vi "Periodic Tasks.vi"() -> ()   [LabVIEW 2011]
doc: "This VI runs in parallel to other tasks. It can contain as many user-defined periodic loops as you need. These can carry out PID or other sorts of timed response."
uses:
  <vilib>/Rock Robotics/SystemInterfaces/Utilities/FPGA_UtilitiesLED State.ctl
  <vilib>/Rock Robotics/SystemInterfaces/Utilities/FPGA_UtilitiesLED Source.ctl
  Robot Global Data.vi
  <vilib>/Rock Robotics/WPI/Relay/WPI_RelayValue.ctl
panel:
  out "Both Hit?":bool
  out "Desired Ramp POT Voltage":dbl
  out "Ramp POT Angle":dbl
  out "Ramp Pot Voltage":dbl
  out "ON/OFF":bool
  out "Rate 3":dbl
  out "error out 4":errorcluster
  out "Direction 3":bool
  out "Distance 3":dbl
  out "Distance 2":dbl
  out "Direction 2":bool
  out "error out 3":errorcluster
  out "Rate 2":dbl
  out "Rate":dbl
  out "error out 2":errorcluster
  out "I2C":bool
  out "Angular Rate":dbl
  out "Angle":dbl
  out "Direction":bool
  out "Distance":dbl
  # "Speed to move to home"
  # "Target Tracking"
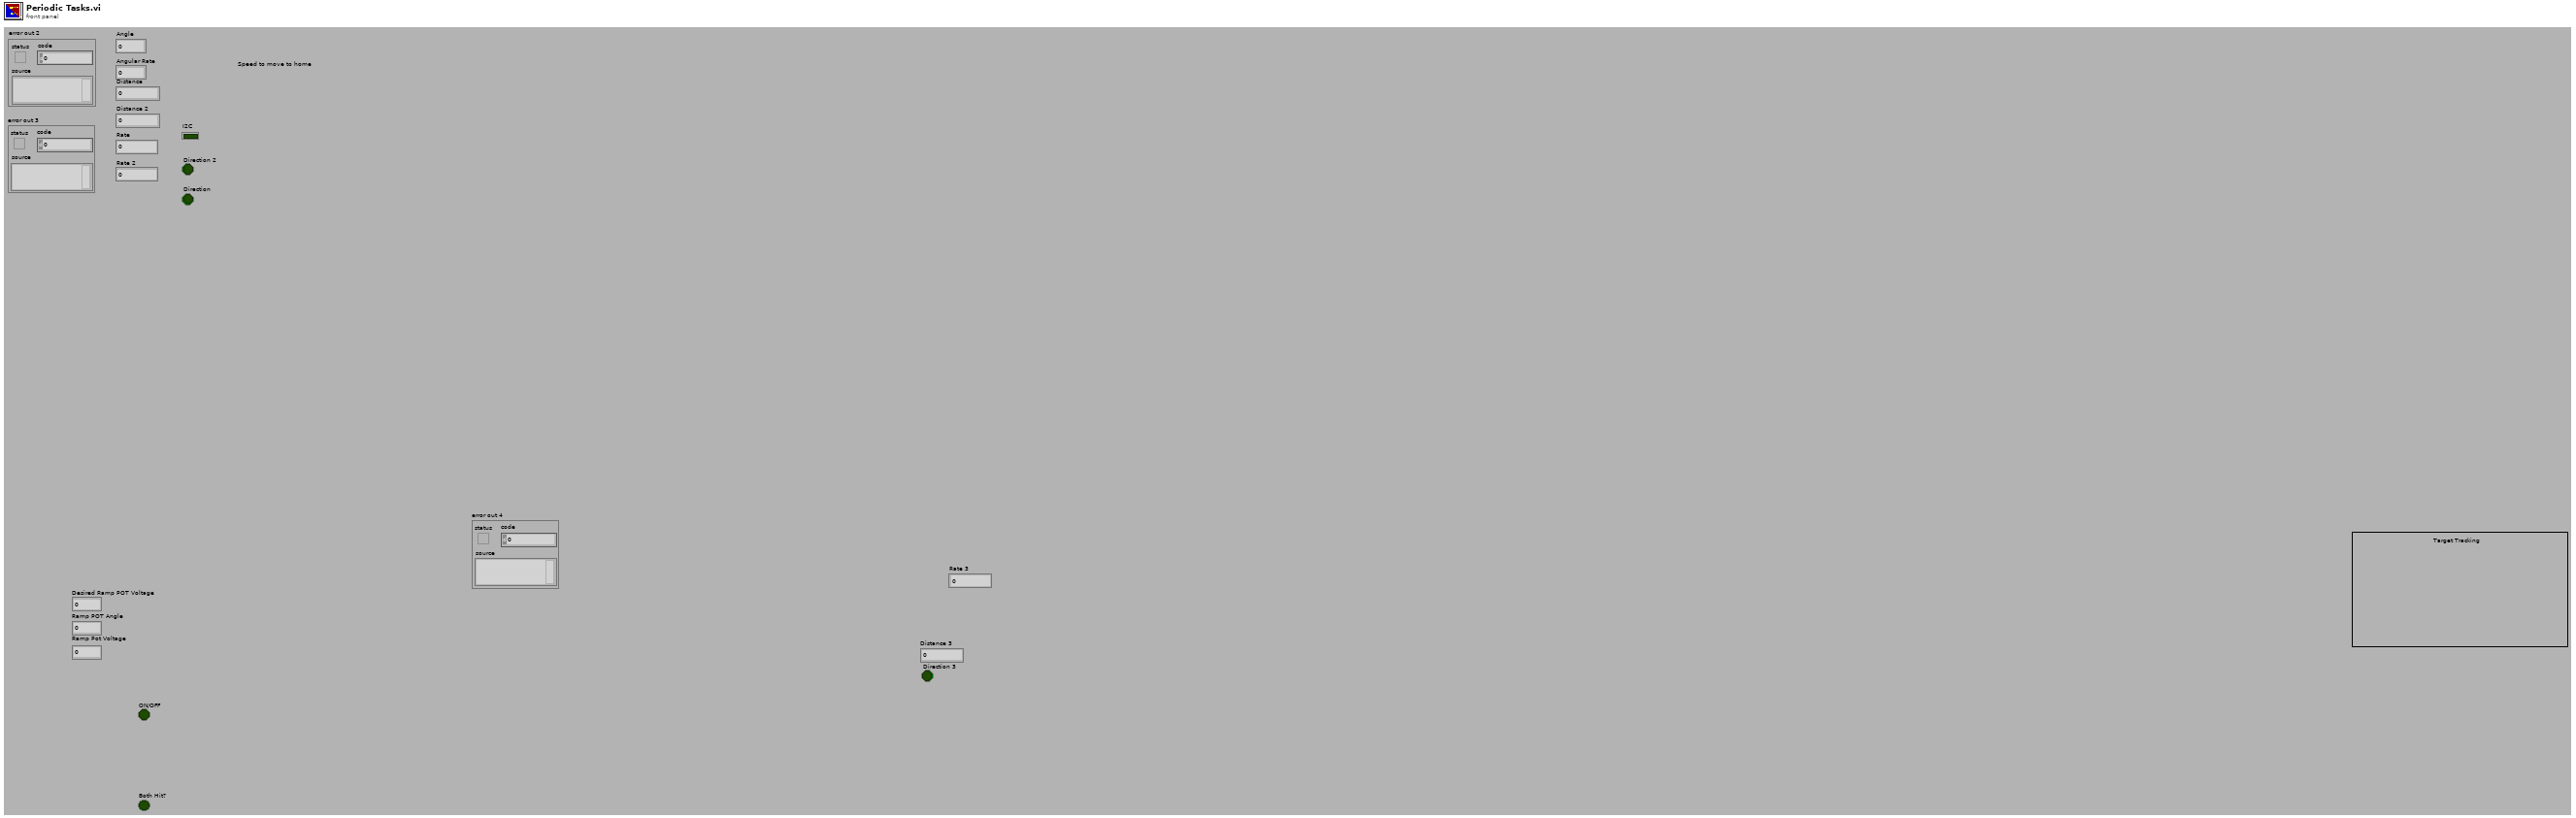
[diagram p1: front panel]
types:
  T1 = typedef "WPI_EncoderDevRef.ctl" = cluster{"DevStatus":errorcluster, "EncoderIndex":T2, "CounterIndex":T3, "DistancePerCount":dbl, "Decoding Type":T4}
  T2 = typedef "FPGA_EncoderIdx.ctl" = enum8{"Enc 0", "Enc 1", "Enc 2", "Enc 3", "Invalid"}
  T3 = typedef "FPGA_CounterCtrSystemIndex.ctl" = enum8{"Ctr 0", "Ctr 1", "Ctr 2", "Ctr 3", "Ctr 4", "Ctr 5", "Ctr 6", "Ctr 7", "Invalid"}
  T4 = typedef "WPI_EncoderType.ctl" = enum16{"1x", "2x", "4x"}
  T5 = typedef "WPI_RelayValue.ctl" = enum16{"Off", "On", "Forward", "Reverse"}
  T6 = typedef "WPI_AnalogChannelDevRef.ctl" = cluster{"DevStatus":errorcluster, "Analog Module":T7, "Analog Channel":T8}
  T7 = typedef "FPGA_TypedefAnalogModule.ctl" = enum16{"Analog Module 1", "Analog Module 2"}
  T8 = typedef "FPGA_AIChannel.ctl" = enum8{"AI 1", "AI 2", "AI 3", "AI 4", "AI 5", "AI 6", "AI 7", "AI 8", "Invalid"}
  T9 = typedef "WPI_RelayDevRef.ctl" = cluster{"DevStatus":errorcluster, "Relay Channel":T10, "Digital Module":T11, "Relay Direction":T12}
  T10 = typedef "FPGA_DIORelayChannel.ctl" = enum8{"Relay 1", "Relay 2", "Relay 3", "Relay 4", "Relay 5", "Relay 6", "Relay 7", "Relay 8", "Invalid"}
  T11 = typedef "FPGA_TypedefDigitalModule.ctl" = enum16{"Digital Module 1", "Digital Module 2"}
  T12 = typedef "WPI_RelayDirection.ctl" = enum16{"Both directions", "Forward only", "Reverse only"}
  T13 = typedef "WPI_GyroDevRef.ctl" = cluster{"DevStatus":errorcluster, "Analog Module":T7, "Analog Channel":T8, "Offset":dbl, "Gain (VoltsPerDegree/Second)":dbl}
  T14 = typedef "WPI_JoystickDevRef.ctl" = cluster{"Device":T15}
  T15 = typedef "WPI_JoystickDeviceEnum.ctl" = enum16{"USB 1", "USB 2", "USB 3", "USB 4", "Kinect 1", "Kinect 2"}
  T16 = cluster{"axis 1 (x)":dbl, "axis 2 (y)":dbl, "axis 3 (throttle)":dbl, "axis 4":dbl, "axis 5":dbl, "axis 6":dbl}
  T17 = typedef "WPI_JoystickButtonState.ctl" = cluster{"Button 1":bool, "Button 2":bool, "Button 3":bool, "Button 4":bool, "Button 5":bool, "Button 6":bool, "Button 7":bool, "Button 8":bool, "Button 9":bool, "Button 10":bool, "Button 11":bool, "Button 12":bool}
  T18 = typedef "WPI_MotorControlDeviceRef.ctl" = cluster{"DeviceStatus":errorcluster, "Type":enum16{"PWM", "CAN"}, "PWM":cluster{"Digital Module":T11, "PWM Channel":T19, "DeadBand":T20}, "CAN":cluster{"Device Number":u8, "Control Mode":T21, "Semaphore":T22, "Max Vout":dbl}, "Invert":bool, "TransformRef":T23, "InvTransformRef":T23}
  T19 = typedef "FPGA_DIOPWMChannel.ctl" = enum8{"PWM 1", "PWM 2", "PWM 3", "PWM 4", "PWM 5", "PWM 6", "PWM 7", "PWM 8", "PWM 9", "PWM 10", "Invalid"}
  T20 = typedef "WPI_PWMDeadband.ctl" = cluster{"Name":string, "maxPositivePwm":i32, "minPositivePwm":i32, "centerPwm":i32, "maxNegativePwm":i32, "minNegativePwm":i32, "angularRange":u16}
  T21 = typedef "WPI_CANJaguar_ControlMode.ctl" = enum8{"Percent VBus", "Current", "Speed", "Position", "Voltage"}
  T22 = typedef "Semaphore RefNum" = refnum<k1>
  T23 = typedef "WPI_PWMTransform_ConPane.ctl" = refnum<vi>
  T24 = cluster{"Driver Station Digital Output (1-8)[0]":bool, "Driver Station Digital Output (1-8)[1]":bool, "Driver Station Digital Output (1-8)[2]":bool, "Driver Station Digital Output (1-8)[3]":bool, "Driver Station Digital Output (1-8)[4]":bool, "Driver Station Digital Output (1-8)[5]":bool, "Driver Station Digital Output (1-8)[6]":bool, "Driver Station Digital Output (1-8)[7]":bool, "Driver Station Digital Output (1-8)[8]":bool}
  T25 = typedef "FPGA_UtilitiesLED State.ctl" = enum16{"Off", "On", "Toggle"}
  T26 = typedef "FPGA_UtilitiesLED Source.ctl" = enum16{"User LED", "FPGA LED"}
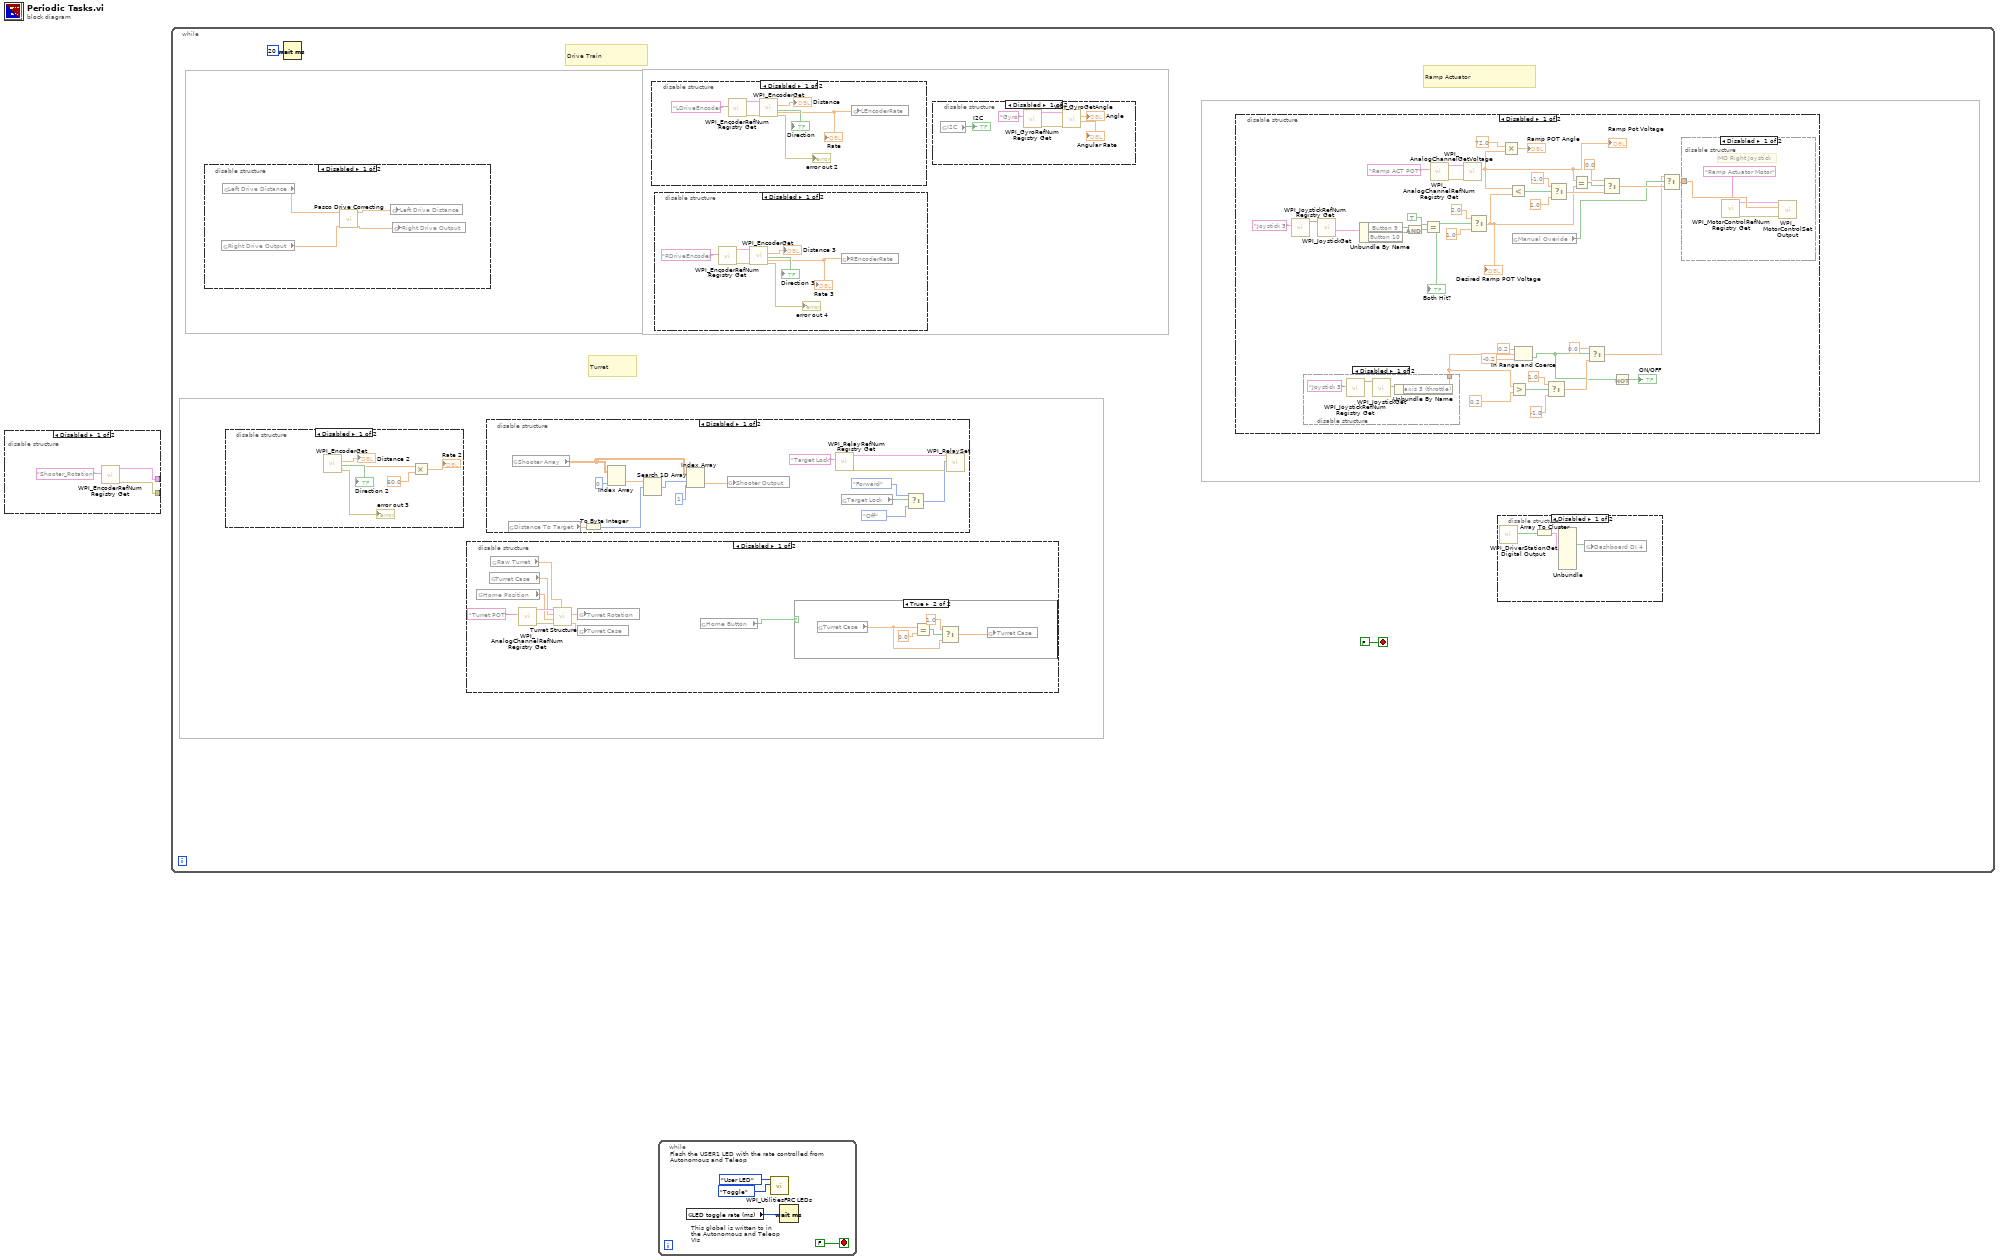
[diagram p0: block diagram]
diagram:
  n1 = disable-structure shown="Disabled" {
    disable-tunnel: [w2 _] -> _
    disable-tunnel: [w1 _] -> _
    frame Disabled {
      n2 = call <vilib>:"WPI_EncoderRefNum Registry Get.vi"("refnum name"="Shooter_Rotation") -> ("error out"=w2:errorcluster, "EncoderDevRef"=w1:T1)  [unwired: 9 in]
    }
    frame Enabled {
    }
  }
  n3 = while {
    stop <- FALSE stop-if-true
    # "Turret"
    # "Drive Train"
    # "Ramp Actuator"
    n4 = disable-structure shown="Disabled" {
      frame Disabled {
        n5 = global read "Robot Global Data.vi" "Right Drive Output"() -> (w8:dbl)
        n6 = global read "Robot Global Data.vi" "Left Drive Distance"() -> (w9:dbl)
        n7 = call "Pasco Drive Correcting.vi"("RightDriveOutput"=w8, "LeftDriveOutput"=w9) -> ("RightDriveOutput"=w6:dbl, "LeftDriveOutput"=w7:dbl)  [unwired: 8 in]
        n8 = global write "Robot Global Data.vi" "Left Drive Distance"(w7) -> ()
        n9 = global write "Robot Global Data.vi" "Right Drive Output"(w6) -> ()
      }
      frame Enabled {
      }
    }
    n10 = disable-structure shown="Disabled" {
      frame Disabled {
        n11 = call <vilib>:"WPI_EncoderGet.vi"() -> ("error out"=→"error out 3":errorcluster, "Direction"=→"Direction 2":bool, "Distance"=→"Distance 2":dbl, "Rate"=w94:dbl)  [unwired: 6 in, 2 out]
        n12 = Multiply(x=w94, y=60.0) -> (x*y=→"Rate 2":dbl)
      }
      frame Enabled {
      }
    }
    n13 = Wait (ms)(milliseconds to wait=u32 20) -> ()  [unwired: 1 out]
    n14 = disable-structure shown="Disabled" {
      frame Disabled {
        n15 = global read "Robot Global Data.vi" "Home Position"() -> (w17:dbl)
        n16 = global read "Robot Global Data.vi" "Turret Case"() -> (w18:dbl)
        n17 = global read "Robot Global Data.vi" "Raw Turret"() -> (w16:dbl)
        n18 = call <vilib>:"WPI_AnalogChannelRefNum Registry Get.vi"("refnum name"="Turret POT") -> ("error out"=w19:errorcluster, "AIDeviceRef"=w20:T6)  [unwired: 9 in]
        n19 = call "Turret Structure.vi"("Raw Turret"=w16, "error in (no error)"=w19, "Home postion"=w17, "Turret Case"=w18, "AIDeviceRef"=w20) -> ("Turret Case Output"=w14:dbl, "Turret Output"=w15:dbl)  [unwired: 5 in]
        n20 = global write "Robot Global Data.vi" "Turret Rotation"(w15) -> ()
        n21 = global write "Robot Global Data.vi" "Turret Case"(w14) -> ()
        n22 = global read "Robot Global Data.vi" "Home Button"() -> (w13:bool)
        n23 = case shown="True" w13 {
          frame False {
          }
          frame True {
            n24 = global read "Robot Global Data.vi" "Turret Case"() -> (w23:dbl)
            n25 = Equal?(x=w23, y=0.0) -> (x = y?=w25:bool)
            n26 = Select(t=1.0, s=w25, f=w23) -> (s? t:f=w22:dbl)
            n27 = global write "Robot Global Data.vi" "Turret Case"(w22) -> ()
          }
        }
      }
      frame Enabled {
      }
    }
    n28 = disable-structure shown="Disabled" {
      frame Disabled {
        n29 = global read "Robot Global Data.vi" "Distance To Target"() -> (w104:dbl)
        n30 = global read "Robot Global Data.vi" "Shooter Array"() -> (w102:dbl[][])
        n31 = To Byte Integer(number=w104) -> (8bit integer=w103:i8)
        n32 = Index Array(array=w102, index (col)=0 ("disabled index (col)")) -> (element=w105:dbl[])  [unwired: 1 in]
        n33 = Search 1D Array(1D array=w105, element=w103) -> (index of element=w101:i32)  [unwired: 1 in]
        n34 = Index Array(array=w102, index (row)=w101, index (col)=1 ("disabled index (col)")) -> (element=w99:dbl)
        n35 = global write "Robot Global Data.vi" "Shooter Output"(w99) -> ()
        n36 = call <vilib>:"WPI_RelayRefNum Registry Get.vi"("refnum name"="Target Lock") -> ("error out"=w107:errorcluster, "RelayDevRef"=w108:T9)  [unwired: 9 in]
        n37 = global read "Robot Global Data.vi" "Target Lock"() -> (w113:bool)
        n38 = Select(t=WPI_RelayValue."Forward" ("RelayValue"), s=w113, f=WPI_RelayValue."Off" ("RelayValue")) -> (s? t:f=w110:T5)
        n39 = call <vilib>:"WPI_RelaySet.vi"("error in (no error)"=w107, "RelayValue"=w110, "RelayDevRef"=w108) -> ()  [unwired: 7 in, 2 out]
      }
      frame Enabled {
      }
    }
    n40 = disable-structure shown="Disabled" {
      frame Disabled {
        n41 = call <vilib>:"WPI_EncoderRefNum Registry Get.vi"("refnum name"="LDriveEncoder") -> ("error out"=w84:errorcluster, "EncoderDevRef"=w83:T1)  [unwired: 9 in]
        n42 = call <vilib>:"WPI_EncoderGet.vi"("error in (no error)"=w84, "EncoderDevRef"=w83) -> ("error out"=→"error out 2":errorcluster, "Direction"=→"Direction":bool, "Distance"=→"Distance":dbl, "Rate"=w80:dbl)  [unwired: 4 in, 2 out]
        "Rate" <- w80
        n43 = global write "Robot Global Data.vi" "LEncoderRate"(w80) -> ()
      }
      frame Enabled {
      }
    }
    n44 = disable-structure shown="Disabled" {
      frame Disabled {
        n45 = call <vilib>:"WPI_EncoderRefNum Registry Get.vi"("refnum name"="RDriveEncoder") -> ("error out"=w77:errorcluster, "EncoderDevRef"=w76:T1)  [unwired: 9 in]
        n46 = call <vilib>:"WPI_EncoderGet.vi"("error in (no error)"=w77, "EncoderDevRef"=w76) -> ("error out"=→"error out 4":errorcluster, "Direction"=→"Direction 3":bool, "Distance"=→"Distance 3":dbl, "Rate"=w73:dbl)  [unwired: 4 in, 2 out]
        "Rate 3" <- w73
        n47 = global write "Robot Global Data.vi" "REncoderRate"(w73) -> ()
      }
      frame Enabled {
      }
    }
    n48 = disable-structure shown="Disabled" {
      frame Disabled {
        n49 = global read "Robot Global Data.vi" "I2C"() -> (→"I2C":bool)
        n50 = call <vilib>:"WPI_GyroRefNum Registry Get.vi"("refnum name"="Gyro") -> ("error out"=w91:errorcluster, "GyroDevRef"=w92:T13)  [unwired: 9 in]
        n51 = call <vilib>:"WPI_GyroGetAngle.vi"("error in (no error)"=w91, "GyroDevRef"=w92) -> ("Angular Rate"=→"Angular Rate":dbl, "Angle"=→"Angle":dbl)  [unwired: 6 in, 2 out]
      }
      frame Enabled {
      }
    }
    n52 = disable-structure shown="Disabled" {
      frame Disabled {
        n53 = call <vilib>:"WPI_JoystickRefNum Registry Get.vi"("refnum name"="Joystick 3") -> ("JoystickDevRef"=w62:T14)  [unwired: 9 in, 1 out]
        n54 = disable-structure shown="Disabled" {
          disable-tunnel: [w69 _] -> w33
          frame Disabled {
            n55 = call <vilib>:"WPI_JoystickRefNum Registry Get.vi"("refnum name"="Joystick 3") -> ("JoystickDevRef"=w72:T14)  [unwired: 9 in, 1 out]
            n56 = call <vilib>:"WPI_JoystickGet.vi"("JoystickDevRef"=w72) -> ("Axes"=w70:T16)  [unwired: 4 in, 2 out]
            n57 = Unbundle By Name(w70) -> ("axis 3 (throttle)"=w69:dbl)
          }
          frame Enabled {
          }
        }
        n58 = call <vilib>:"WPI_JoystickGet.vi"("JoystickDevRef"=w62) -> ("Buttons"=w64:T17)  [unwired: 4 in, 2 out]
        n59 = Unbundle By Name(w64) -> ("Button 9"=w61:bool, "Button 10"=w60:bool)
        n60 = And(x=w61, y=w60) -> (x .and. y?=w59:bool)
        n61 = Equal?(x=TRUE, y=w59) -> (x = y?=w54:bool)
        "Both Hit?" <- w54
        n62 = call <vilib>:"WPI_AnalogChannelRefNum Registry Get.vi"("refnum name"="Ramp ACT POT") -> ("error out"=w57:errorcluster, "AIDeviceRef"=w56:T6)  [unwired: 9 in]
        n63 = call <vilib>:"WPI_AnalogChannelGetVoltage.vi"("error in (no error)"=w57, "AIDeviceRef"=w56) -> ("Voltage"=w44:dbl)  [unwired: 7 in, 2 out]
        "Ramp Pot Voltage" <- w44
        n64 = Select(t=2.0, s=w54, f=1.0 ("t")) -> (s? t:f=w47:dbl)
        "Desired Ramp POT Voltage" <- w47
        n65 = Multiply(x=72.0, y=w44) -> (x*y=→"Ramp POT Angle":dbl)
        n66 = Less?(x=w44, y=w47) -> (x < y?=w51:bool)
        n67 = Greater?(x=w33, y=0.2) -> (0:w34:bool)
        n68 = global read "Robot Global Data.vi" "Manual Overide"() -> (w40:bool)
        n69 = In Range and Coerce(upper limit=0.2, x=w33, lower limit=-0.2) -> (In Range?=w28:bool)  [unwired: 1 out]
        n70 = Select(t=1.0, s=w34, f=-1.0) -> (s? t:f=w35:dbl)
        n71 = Select(t=-1.0, s=w51, f=1.0) -> (s? t:f=w50:dbl)
        n72 = Equal?(x=w44, y=w47) -> (x = y?=w53:bool)
        n73 = Select(t=0.0, s=w28, f=w35) -> (s? t:f=w29:dbl)
        n74 = Select(t=0.0, s=w53, f=w50) -> (s? t:f=w41:dbl)
        n75 = Not(x=w28) -> (.not. x?=→"ON/OFF":bool)
        n76 = Select(t=w29, s=w40, f=w41) -> (s? t:f=w39:dbl)
        n77 = disable-structure shown="Disabled" {
          disable-tunnel: w39 -> [w67 _]
          frame Disabled {
            # "MO Right Joystick"
            n78 = call <vilib>:"WPI_MotorControlRefNum Registry Get.vi"("refnum name"="Ramp Actuator Motor") -> ("error out"=w68:errorcluster, "MotorControlDevRef"=w66:T18)  [unwired: 9 in]
            n79 = call <vilib>:"WPI_MotorControlSetOutput.vi"("error in (no error)"=w68, "Output"=w67, "MotorControlDevRef"=w66) -> ()  [unwired: 7 in, 2 out]
          }
          frame Enabled {
          }
        }
      }
      frame Enabled {
      }
    }
    n80 = disable-structure shown="Disabled" {
      frame Disabled {
        n81 = call <vilib>:"WPI_DriverStationGet Digital Output.vi"() -> ("Driver Station Digital Output (1-8)"=w12:bool[])  [unwired: 10 in, 1 out]
        n82 = Array To Cluster(array=w12) -> (cluster=w11:T24)
        n83 = Unbundle(w11) -> ("Driver Station Digital Output (1-8)[3]"=w10:bool)  [unwired: 8 out]
        n84 = global write "Robot Global Data.vi" "Dashboard DI 4"(w10) -> ()
      }
      frame Enabled {
      }
    }
  }
  n85 = while {
    stop <- FALSE stop-if-true
    # "This global is written to in the Autonomous and Teleop VIs"
    # "Flash the USER1 LED with the rate controlled from Autonomous and Teleop"
    n86 = global read "Robot Global Data.vi" "LED toggle rate (ms)"() -> (w114:u32)
    n87 = call <vilib>:"WPI_UtilitiesFRC LEDs.vi"("State"=FPGA_UtilitiesLED_State."Toggle", "LED Type"=FPGA_UtilitiesLED_Source."User LED") -> ()  [unwired: 1 in, 9 out]
    n88 = Wait (ms)(milliseconds to wait=w114) -> ()  [unwired: 1 out]
  }
